vi "Scan Control View.vi"(10 "User Events in":refnum<class "User Events.lvclass">) -> ()   [LabVIEW 2015, in "FAMT Views.lvlib"]
uses:
  FAMT Views.lvlib
  Typedefs/WaveformTypes.ctl
  User Events/User Events.lvclass
  Commands/Command Factory/Command Factory.lvclass
  User Events/User Events.lvclass/User Events.ctl
  Typedefs/StateTypes.ctl
  Typedefs/ScanSettings.ctl
  Typedefs/WaveformSettings.ctl
  Commands/Start Scan Command/Start Scan Command.lvclass
  Commands/Start Scan Command/Start Scan Command.lvclass/Start Scan Command.ctl
  Typedefs/ActuatorTypes.ctl
  Typedefs/FAMT Typedefs.lvlib
panel:
  in  "Scan Name":string
  in  "Test Stand Serial Number":string
  in  "Actuator Serial Number":string
  in  "Lateral Waveform":T2={"Waveform"=enum."Sine", "Amplitude"=1.0, "Settling Time"=1.0, "Offset"=0.0, "Delay"=0.0, "Frequency"=2.0, "F1"=1.0, "F2"=10.0, "Duty Cycle"=0.5, "Ramp Time"=1.0, "Hold Time"=2.0} {"Delay" min=0.0 max=1.0 format="%.3f"; "Duty Cycle" min=0.0 max=1.0; "Offset" min=0.0 max=1.0 format="%.3f"; "Amplitude" min=0.0 max=1.0 format="%.3f"}
  in  "Axial Waveform":T2={"Waveform"=enum."Sine", "Amplitude"=1.0, "Settling Time"=1.0, "Offset"=0.0, "Delay"=0.0, "Frequency"=2.0, "F1"=1.0, "F2"=10.0, "Duty Cycle"=0.5, "Ramp Time"=1.0, "Hold Time"=2.0} {"Delay" min=0.0 max=1.0 format="%.3f"; "Duty Cycle" min=0.0 max=1.0; "Offset" min=0.0 max=1.0 format="%.3f"; "Amplitude" min=0.0 max=1.0 format="%.3f"}
  in  "Notes":string
  in  "Test Name":string
  in  "Operator":string
  in  "Samples":u32=1000 caption="s"
  in  "startScan":bool
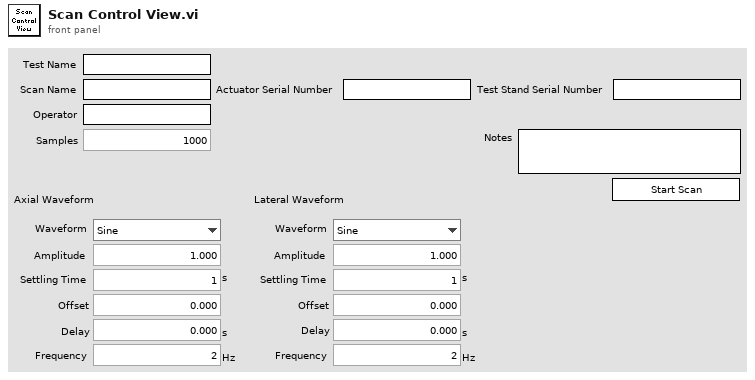
[diagram p1: front panel]
types:
  T1 = typedef "FAMT Typedefs.lvlib/WaveformTypes.ctl" = enum16{"Sine", "Triangle", "Square", "Sawtooth", "Chirp", "Gaussian", "Trapezoid", "Constant"}
  T2 = cluster{"Waveform":T1, "Amplitude":dbl, "Settling Time":dbl[unit], "Offset":dbl, "Delay":dbl[unit], "Frequency":dbl[unit], "F1":dbl[unit], "F2":dbl[unit], "Duty Cycle":dbl, "Ramp Time":dbl[unit], "Hold Time":dbl[unit]}
  T3 = typedef "FAMT Typedefs.lvlib/Publish Data Events.ctl" = cluster{"State":refnum<user-event>, "ErrorCode":refnum<user-event>, "Scan Progress":refnum<user-event>}
  T4 = typedef "FAMT Typedefs.lvlib/Subscribe Data Events.ctl" = cluster{"Command":refnum<user-event>}
  T5 = cluster{"Event Registration Refnum":refnum<event-registration>, "Event Registration Refnum":refnum<event-registration>}
  T6 = typedef "FAMT Typedefs.lvlib/StateTypes.ctl" = enum16{"Offline State", "Fault State", "Standby State", "Disabled State", "Enabled State", "Wait For User Input State", "Perform Scan State"}
  T7 = typedef "FAMT Typedefs.lvlib/WaveformSettings.ctl" = cluster{"Sample Count":u32, "Amplitude":dbl, "Offset":dbl, "Frequency":dbl[unit], "Waveform":T1, "F1":dbl[unit], "F2":dbl[unit], "Duty Cycle":dbl, "ILC Rate":dbl[unit], "Ramp Time":dbl[unit], "Hold Time":dbl[unit], "Settling Time":dbl[unit], "Delay":dbl[unit]}
  T8 = typedef "FAMT Typedefs.lvlib/ScanSettings.ctl" = cluster{"Operator":string, "Scan Name":string, "Notes":string, "Axial Settings":T7, "Lateral Settings":T7, "Actuator Serial Number":string, "Test Stand Serial Number":string, "Test Name":string}
  T9 = typedef "FAMT Typedefs.lvlib/ActuatorTypes.ctl" = enum16{"Single", "Dual"}
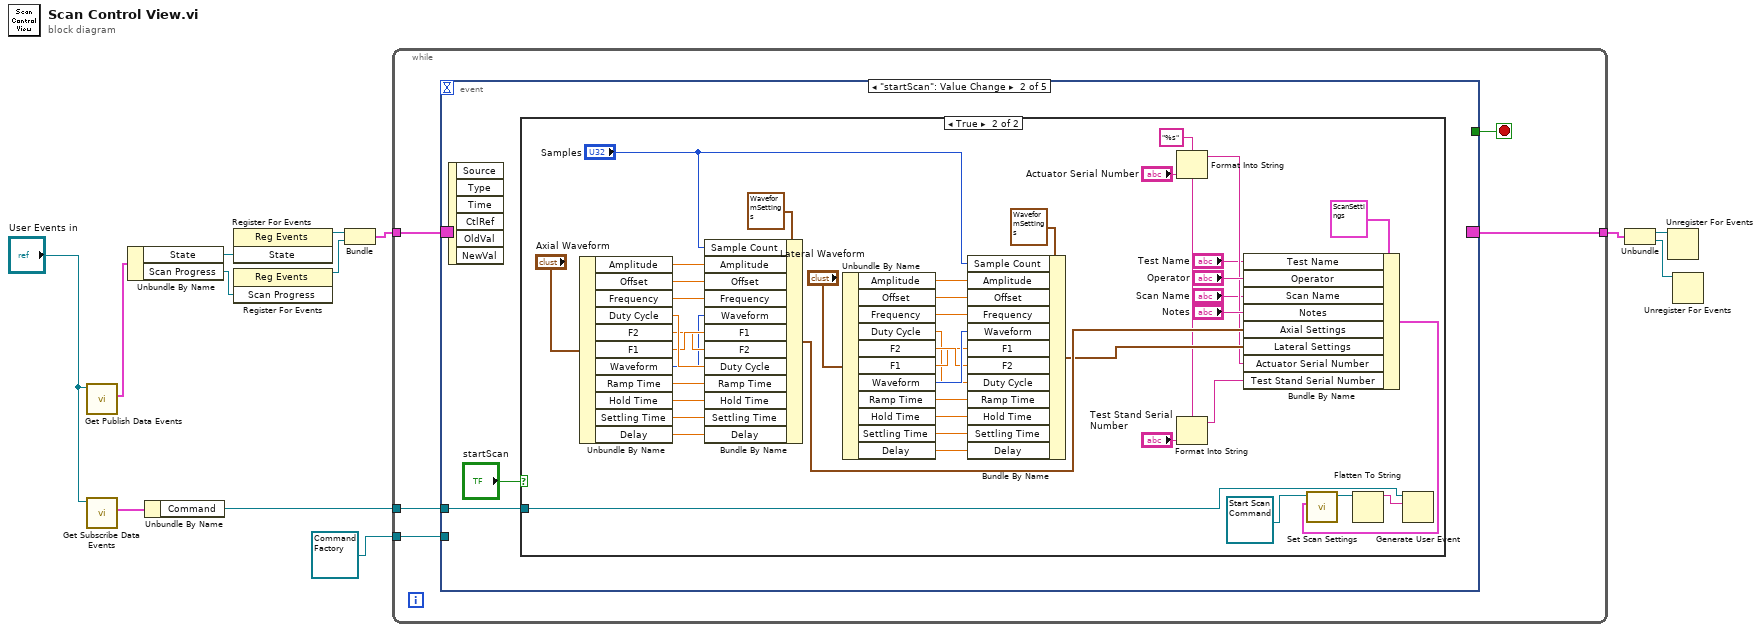
[diagram p0: block diagram]
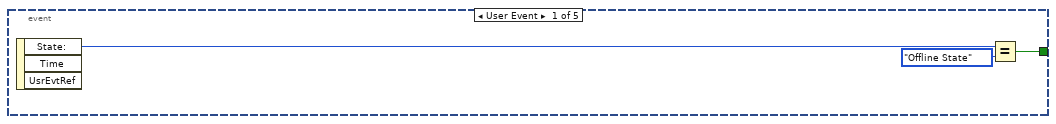
[diagram p2: hidden frame]
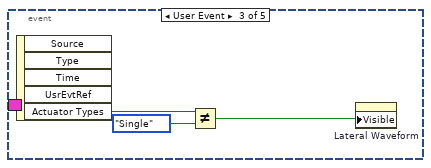
[diagram p4: hidden frame]
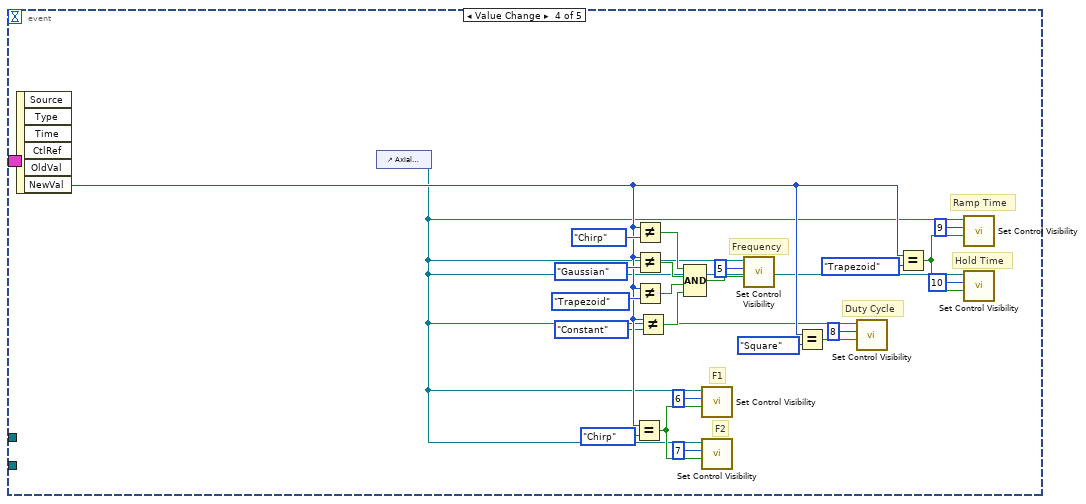
[diagram p5: hidden frame]
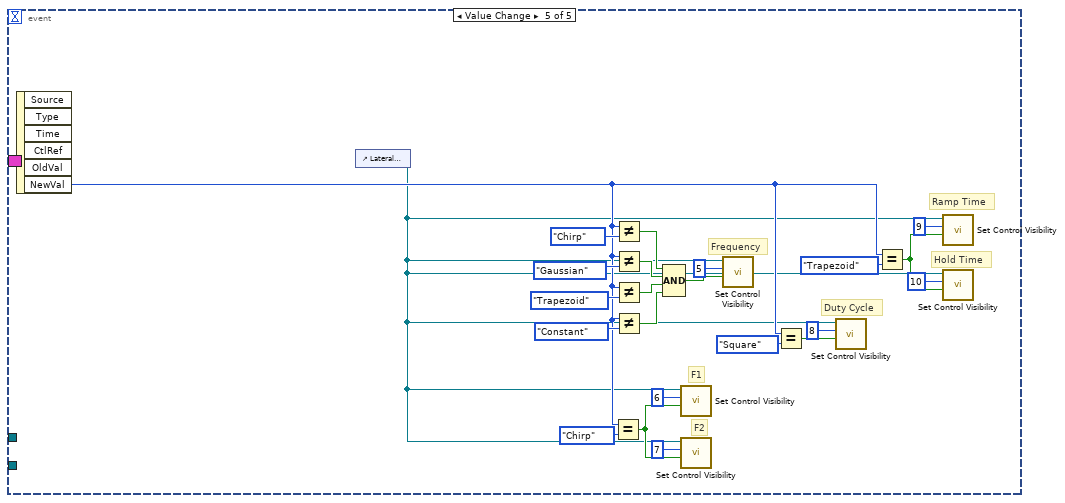
[diagram p6: hidden frame]
diagram:
  n1 = call "Get Publish Data Events.vi"("UserEvents in"="User Events in") -> ("Publish Data Events"=w13:T3)  [unwired: 9 in, 1 out]
  n2 = call "Get Subscribe Data Events.vi"("UserEvents in"="User Events in") -> ("Subscribe Data Events"=w7:T4)  [unwired: 9 in, 1 out]
  n3 = Unbundle By Name(w13) -> ("State"=w12:refnum<user-event>, "Scan Progress"=w3:refnum<user-event>)
  n4 = Unbundle By Name(w7) -> ("Command"=w5:refnum<user-event>)
  n5 = register-events(w12) -> (reference out=w11:refnum<event-registration>)  [unwired: 2 in, 1 out]
  n6 = register-events(w3) -> (reference out=w2:refnum<event-registration>)  [unwired: 2 in, 1 out]
  n7 = Bundle("Event Registration Refnum"=w11, "Event Registration Refnum"=w2) -> (w8:T5)  [unwired: 1 in]
  n8 = while {
    tunnel: w8 -> [w18]
    tunnel: [w17] -> w9
    tunnel: w5 -> [w15]
    tunnel: refnum<class "Command Factory.lvclass"> refnum ("CommandFactory.lvclass") -> [w14]
    stop <- w16 stop-if-true
    n9 = event shown="[1] \"startScan\": Value Change" {
      selector: w18 -> [_ _ _ _ _]
      dyn-events: [_ _ _ _ _] -> w17
      timeout: _ -> [_ _ _ _ _]
      tunnel: [w20 _ _ _ _] -> w16
      tunnel: w15 -> [_ w22 _ _ _]
      tunnel: w14 -> [_ _ _ _ _]
      event User Event {
        n10 = event-data() -> ("State:"=w19:T6)  [unwired: 1 in, 2 out]
        n11 = Equal?(x=w19, y=StateTypes."Offline State") -> (x = y?=w20:bool)
      }
      event "startScan": Value Change {
        n12 = event-data() -> ()  [unwired: 1 in, 6 out]
        n13 = case shown="True" "startScan" {
          tunnel: w22 -> [_ w66]
          frame False {
          }
          frame True {
            w29 = "%s"
            n14 = Unbundle By Name("Axial Waveform") -> ("Amplitude"=w61:dbl, "Offset"=w60:dbl, "Frequency"=w59:dbl[unit], "Duty Cycle"=w58:dbl, "F2"=w56:dbl[unit], "F1"=w57:dbl[unit], "Waveform"=w55:T1, "Ramp Time"=w54:dbl[unit], "Hold Time"=w53:dbl[unit], "Settling Time"=w52:dbl[unit], "Delay"=w51:dbl[unit])
            n15 = Bundle By Name(cluster=T7 {"Sample Count"=0, "Amplitude"=0.0, "Offset"=0.0, "Frequency"=0.0, "Waveform"=enum."Sine", "F1"=0.0, "F2"=0.0, "Duty Cycle"=0.0, "ILC Rate"=0.0, "Ramp Time"=0.0, "Hold Time"=0.0, "Settling Time"=0.0, "Delay"=0.0} ("Waveform Settings"), "Sample Count"="Samples", "Amplitude"=w61, "Offset"=w60, "Frequency"=w59, "Waveform"=w55, "F1"=w57, "F2"=w56, "Duty Cycle"=w58, "Ramp Time"=w54, "Hold Time"=w53, "Settling Time"=w52, "Delay"=w51) -> (w33:T7)
            n16 = Unbundle By Name("Lateral Waveform") -> ("Amplitude"=w40:dbl, "Offset"=w41:dbl, "Frequency"=w42:dbl[unit], "Duty Cycle"=w43:dbl, "F2"=w45:dbl[unit], "F1"=w44:dbl[unit], "Waveform"=w46:T1, "Ramp Time"=w47:dbl[unit], "Hold Time"=w48:dbl[unit], "Settling Time"=w49:dbl[unit], "Delay"=w50:dbl[unit])
            n17 = Bundle By Name(cluster=T7 {"Sample Count"=0, "Amplitude"=0.0, "Offset"=0.0, "Frequency"=0.0, "Waveform"=enum."Sine", "F1"=0.0, "F2"=0.0, "Duty Cycle"=0.0, "ILC Rate"=0.0, "Ramp Time"=0.0, "Hold Time"=0.0, "Settling Time"=0.0, "Delay"=0.0} ("Waveform Settings"), "Sample Count"="Samples", "Amplitude"=w40, "Offset"=w41, "Frequency"=w42, "Waveform"=w46, "F1"=w44, "F2"=w45, "Duty Cycle"=w43, "Ramp Time"=w47, "Hold Time"=w48, "Settling Time"=w49, "Delay"=w50) -> (w32:T7)
            n18 = Format Into String(format string=w29, "Actuator Serial Number") -> (resulting string=w26:string)  [unwired: 2 in, 1 out]
            n19 = Format Into String(format string=w29, "Test Stand Serial Number") -> (resulting string=w27:string)  [unwired: 2 in, 1 out]
            n20 = Bundle By Name(cluster=T8 {"Operator"="", "Scan Name"="", "Notes"="", "Axial Settings"={"Sample Count"=0, "Amplitude"=0.0, "Offset"=0.0, "Frequency"=0.0, "Waveform"=enum."Sine", "F1"=0.0, "F2"=0.0, "Duty Cycle"=0.0, "ILC Rate"=0.0, "Ramp Time"=0.0, "Hold Time"=0.0, "Settling Time"=0.0, "Delay"=0.0}, "Lateral Settings"={"Sample Count"=0, "Amplitude"=0.0, "Offset"=0.0, "Frequency"=0.0, "Waveform"=enum."Sine", "F1"=0.0, "F2"=0.0, "Duty Cycle"=0.0, "ILC Rate"=0.0, "Ramp Time"=0.0, "Hold Time"=0.0, "Settling Time"=0.0, "Delay"=0.0}, "Actuator Serial Number"="", "Test Stand Serial Number"="", "Test Name"=""} ("Scan Settings"), "Test Name"="Test Name", "Operator"="Operator", "Scan Name"="Scan Name", "Notes"="Notes", "Axial Settings"=w33, "Lateral Settings"=w32, "Actuator Serial Number"=w26, "Test Stand Serial Number"=w27) -> (w36:T8)
            n21 = call "Set Scan Settings.vi"("Scan Settings"=w36, "Start Closed Loop Scan Command in"=refnum<class "Start Scan Command.lvclass"> refnum ("Start Scan Command.lvclass")) -> ("Start Closed Loop Scan Command out"=w65:refnum<class "Start Scan Command.lvclass">)  [unwired: 9 in]
            n22 = Flatten To String(anything=w65) -> (data string=w67:string)  [unwired: 3 in, 2 out]
            n23 = Generate User Event(user event=w66, event data cluster=w67) -> ()  [unwired: 2 in, 2 out]
          }
        }
      }
      event User Event {
        n24 = event-data() -> ("Actuator Types"=w70:T9)  [unwired: 1 in, 4 out]
        n25 = Not Equal?(x=w70, y=ActuatorTypes."Single") -> (x != y?=w68:bool)
        n26 = property on="Lateral Waveform" class="Clust (strict)"("Visible"=w68) -> ()  [unwired: 2 in, 2 out]
      }
      event Value Change {
        # "Hold Time"
        # "Ramp Time"
        # "F1"
        # "F2"
        # "Duty Cycle"
        # "Frequency"
        n27 = event-data() -> ("NewVal"=w73:T1)  [unwired: 1 in, 5 out]
        n28 = control-ref of="Axial Waveform"() -> (w71:refnum<vi>)
        n29 = Equal?(x=w73, y=WaveformTypes."Chirp") -> (x = y?=w79:bool)
        n30 = Not Equal?(x=w73, y=WaveformTypes."Chirp") -> (x != y?=w88:bool)
        n31 = Not Equal?(x=w73, y=WaveformTypes."Gaussian") -> (x != y?=w87:bool)
        n32 = Not Equal?(x=w73, y=WaveformTypes."Trapezoid") -> (x != y?=w75:bool)
        n33 = Not Equal?(x=w73, y=WaveformTypes."Constant") -> (x != y?=w74:bool)
        n34 = Compound Arithmetic op=AND(w88, w87, w75, w74) -> (w77:bool)
        n35 = call "Set Control Visibility.vi"("Visible"=w79, "index"=6, "Waveform"=w71) -> ()  [unwired: 9 in]
        n36 = call "Set Control Visibility.vi"("Visible"=w79, "index"=7, "Waveform"=w71) -> ()  [unwired: 9 in]
        n37 = call "Set Control Visibility.vi"("Visible"=w77, "index"=5, "Waveform"=w71) -> ()  [unwired: 9 in]
        n38 = Equal?(x=w73, y=WaveformTypes."Square") -> (x = y?=w82:bool)
        n39 = call "Set Control Visibility.vi"("Visible"=w82, "index"=8, "Waveform"=w71) -> ()  [unwired: 9 in]
        n40 = Equal?(x=w73, y=WaveformTypes."Trapezoid") -> (x = y?=w85:bool)
        n41 = call "Set Control Visibility.vi"("Visible"=w85, "index"=9, "Waveform"=w71) -> ()  [unwired: 9 in]
        n42 = call "Set Control Visibility.vi"("Visible"=w85, "index"=10, "Waveform"=w71) -> ()  [unwired: 9 in]
      }
      event Value Change {
        # "Hold Time"
        # "Ramp Time"
        # "F1"
        # "F2"
        # "Duty Cycle"
        # "Frequency"
        n43 = event-data() -> ("NewVal"=w96:T1)  [unwired: 1 in, 5 out]
        n44 = control-ref of="Lateral Waveform"() -> (w94:refnum<vi>)
        n45 = Equal?(x=w96, y=WaveformTypes."Chirp") -> (x = y?=w101:bool)
        n46 = Not Equal?(x=w96, y=WaveformTypes."Chirp") -> (x != y?=w111:bool)
        n47 = Not Equal?(x=w96, y=WaveformTypes."Gaussian") -> (x != y?=w110:bool)
        n48 = Not Equal?(x=w96, y=WaveformTypes."Trapezoid") -> (x != y?=w109:bool)
        n49 = Not Equal?(x=w96, y=WaveformTypes."Constant") -> (x != y?=w95:bool)
        n50 = Compound Arithmetic op=AND(w111, w110, w109, w95) -> (w99:bool)
        n51 = call "Set Control Visibility.vi"("Visible"=w101, "index"=6, "Waveform"=w94) -> ()  [unwired: 9 in]
        n52 = call "Set Control Visibility.vi"("Visible"=w101, "index"=7, "Waveform"=w94) -> ()  [unwired: 9 in]
        n53 = call "Set Control Visibility.vi"("Visible"=w99, "index"=5, "Waveform"=w94) -> ()  [unwired: 9 in]
        n54 = Equal?(x=w96, y=WaveformTypes."Square") -> (x = y?=w104:bool)
        n55 = call "Set Control Visibility.vi"("Visible"=w104, "index"=8, "Waveform"=w94) -> ()  [unwired: 9 in]
        n56 = Equal?(x=w96, y=WaveformTypes."Trapezoid") -> (x = y?=w107:bool)
        n57 = call "Set Control Visibility.vi"("Visible"=w107, "index"=9, "Waveform"=w94) -> ()  [unwired: 9 in]
        n58 = call "Set Control Visibility.vi"("Visible"=w107, "index"=10, "Waveform"=w94) -> ()  [unwired: 9 in]
      }
    }
  }
  n59 = Unbundle(w9) -> ("Event Registration Refnum"=w10:refnum<event-registration>, "Event Registration Refnum"=w1:refnum<event-registration>)
  n60 = Unregister For Events(event registration refnum=w10) -> ()  [unwired: 1 in, 1 out]
  n61 = Unregister For Events(event registration refnum=w1) -> ()  [unwired: 1 in, 1 out]
